vi "NewDrive.vi"(2 "Buttons":T1, 3 "Axes":T2) -> (0 "Right Speed":dbl, 1 "Left Speed":dbl)   [LabVIEW 2011]
uses:
  <vilib>/Rock Robotics/WPI/Joystick/WPI_JoystickButtonState.ctl
panel:
  out "number":u32
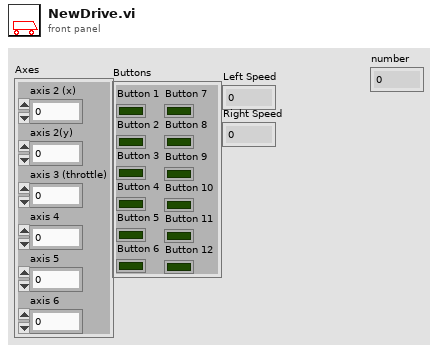
[diagram p1: front panel]
types:
  T1 = typedef "WPI_JoystickButtonState.ctl" = cluster{"Button 1":bool, "Button 2":bool, "Button 3":bool, "Button 4":bool, "Button 5":bool, "Button 6":bool, "Button 7":bool, "Button 8":bool, "Button 9":bool, "Button 10":bool, "Button 11":bool, "Button 12":bool}
  T2 = cluster{"axis 2 (x)":dbl, "axis 2(y)":dbl, "axis 3 (throttle)":dbl, "axis 4":dbl, "axis 5":dbl, "axis 6":dbl}
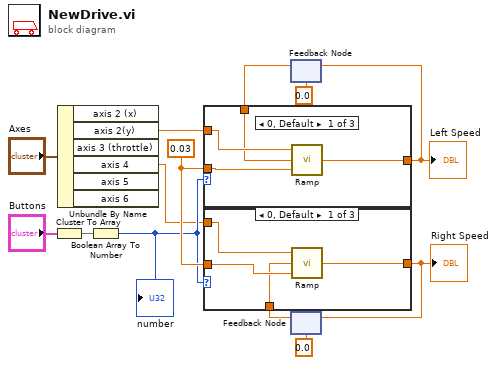
[diagram p0: block diagram]
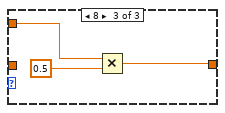
[diagram p3: hidden frame]
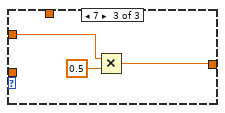
[diagram p5: hidden frame]
diagram:
  w9 = 0.03 ("Speed increment")
  n1 = Cluster To Array(cluster="Buttons") -> (array=w11:bool[])
  n2 = Unbundle By Name("Axes") -> ("axis 2(y)"=w10:dbl, "axis 4"=w1:dbl)  [unwired: 4 out]
  n3 = Boolean Array To Number(Boolean array=w11) -> (number=w2:u32)
  "number" <- w2
  n4 = feedback #1(0.0 ("axis 2(y)")) -> (w5:dbl)
  n5 = case shown="0, Default" w2 {
    tunnel: w10 -> [w17 w18 w21]
    tunnel: w9 -> [w16 _ _]
    tunnel: [w15 w18 w19] -> w4
    tunnel: w5 -> [w14 _ _]
    frame 0, Default {
      n6 = call "Ramp.vi"("Speed increment"=w16, "last speed"=w14, "Joystick speed"=w17) -> ("speed setting"=w15:dbl)
    }
    frame 5 {
    }
    frame 7 {
      n7 = Multiply(x=w21, y=0.5) -> (x*y=w19:dbl)
    }
  }
  "Left Speed" <- w4
  n8 = feedback-in #1(w4) -> ()
  n9 = feedback #2(0.0 ("axis 2(y)")) -> (w6:dbl)
  n10 = case shown="0, Default" w2 {
    tunnel: w1 -> [w25 w26 w29]
    tunnel: w9 -> [w24 _ _]
    tunnel: [w23 w26 w27] -> w3
    tunnel: w6 -> [w22 _ _]
    frame 0, Default {
      n11 = call "Ramp.vi"("Speed increment"=w24, "last speed"=w22, "Joystick speed"=w25) -> ("speed setting"=w23:dbl)
    }
    frame 6 {
    }
    frame 8 {
      n12 = Multiply(x=w29, y=0.5) -> (x*y=w27:dbl)
    }
  }
  "Right Speed" <- w3
  n13 = feedback-in #2(w3) -> ()
